vi "host_global_vars.vi"() -> ()   [LabVIEW 2021]
uses:
  fpga/fpga_dtype_index.ctl
  fpga/fpga_dtype_status.ctl
panel:
  in  "port":u16=8070
  out "server":bool
  out "out of range?":bool
  out "status":T1
  out "cmd paths":path[](array[path])
  out "cmd names":string[](array[string])
  out "form paths":path[](array[path])
  out "form names":string[](array[string])
  out "current command":string
  in  "current values":sgl[](array[numeric])
  in  "index":T2
  out "scan end occurrence":refnum<k4>
  out "data reference":refnum<data-value>
  out "monitor reference":refnum<data-value>
  out "abort":bool
  in  "monitor avg":i32=100
  in  "cmd idx":i32
  out "log_ts file refnum":refnum<file>
  out "log file refnum":refnum<file>
  out "data directory":path
  out "FPGA VI Reference":refnum<k20>
  out "power":bool
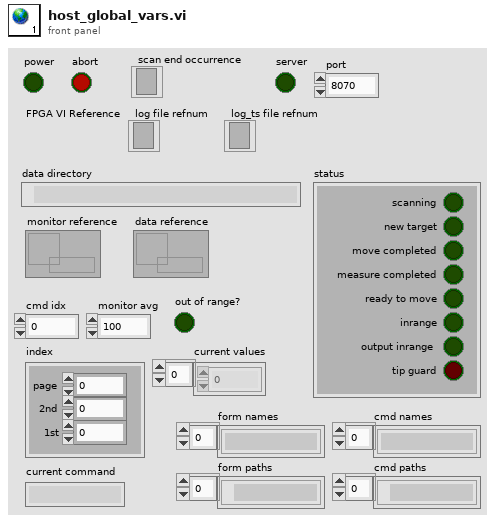
[diagram p1: front panel]
types:
  T1 = typedef "fpga_dtype_status.ctl" = cluster{"scanning":bool, "new target":bool, "move completed":bool, "measure completed":bool, "inrange":bool, "ready to move":bool, "output inrange":bool, "tip guard":bool}
  T2 = typedef "fpga_dtype_index.ctl" = cluster{"page":i16, "2nd":i16, "1st":i16}
diagram:
